vi "TDK 正向工况电流.vi"() -> ()   [LabVIEW 2021]
uses:
  <vilib>/Utility/file.llb/Read Delimited Spreadsheet (DBL).vi
  <instrlib>/TDK-Lambda G Series/TDK-Lambda G Series.lvlib
panel:
  in  "?":enum16{"手动输入", "工况输入"}(ring)
  out "?":bool
  in  "延迟时间":dbl=1.0 caption="延迟时间(s)"
  in  "电流(A)":dbl
  in  "电流方向控制":cluster{"正向":bool, "反向":bool}
  out "工况电流":string[][](table)
  in  "TDK地址":refnum<visa-resource-name>="COM15"
  in  "file path (dialog if empty)":path caption="电流加载"
  in  "电源台数":dbl=3.0
  in  "循环次数":i32
  in  "?":bool
  out "已完成循环次数":i32
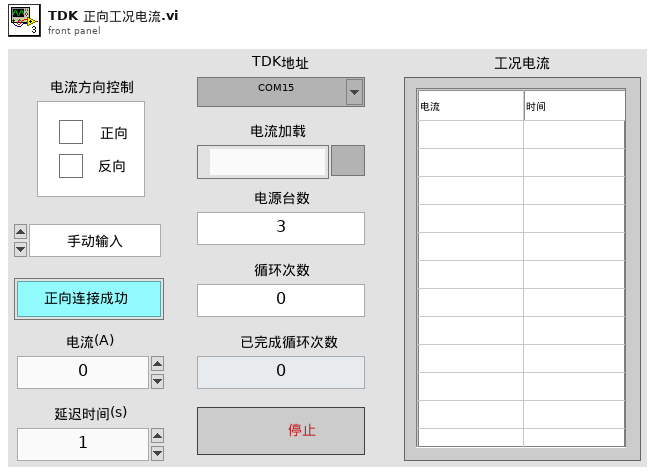
[diagram p1: front panel]
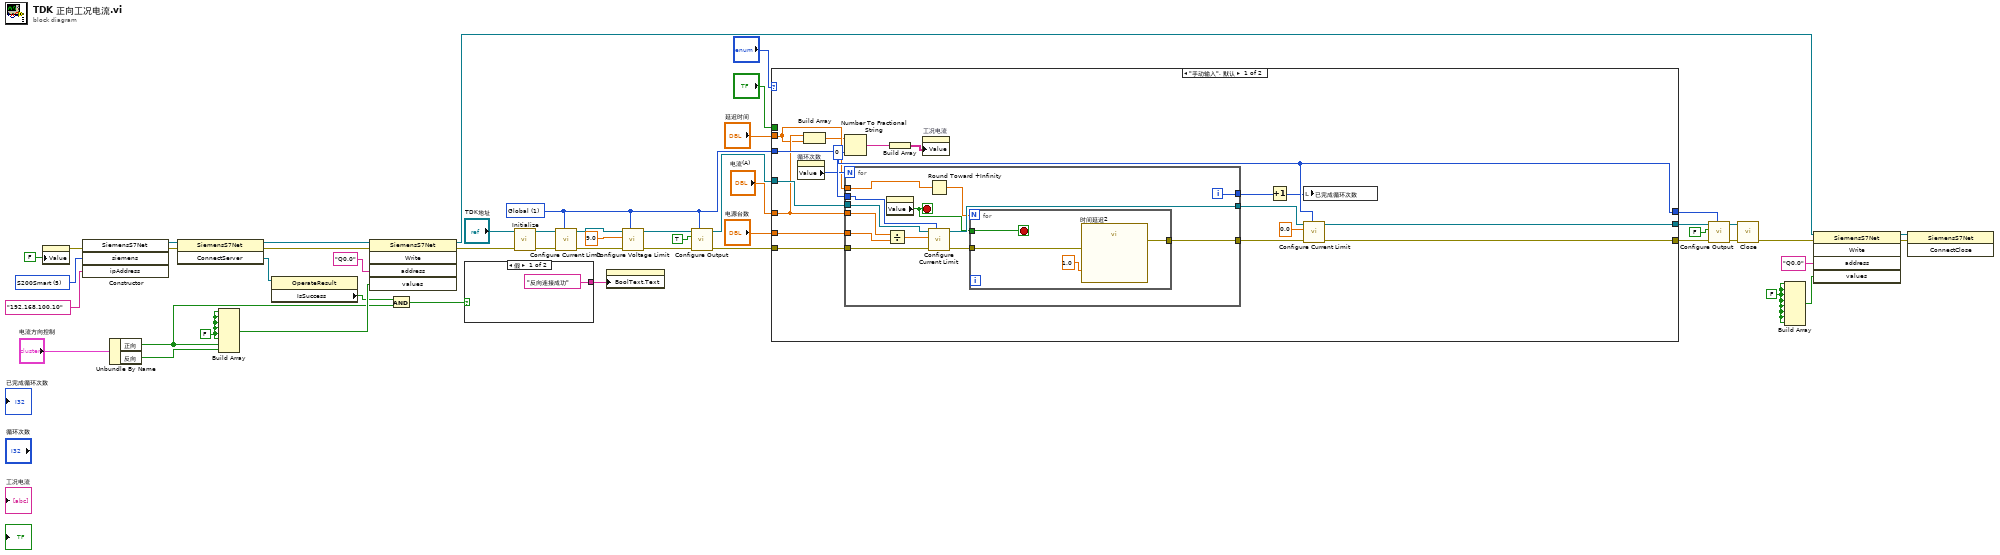
[diagram p0: block diagram]
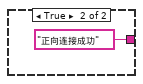
[diagram p2: hidden frame]
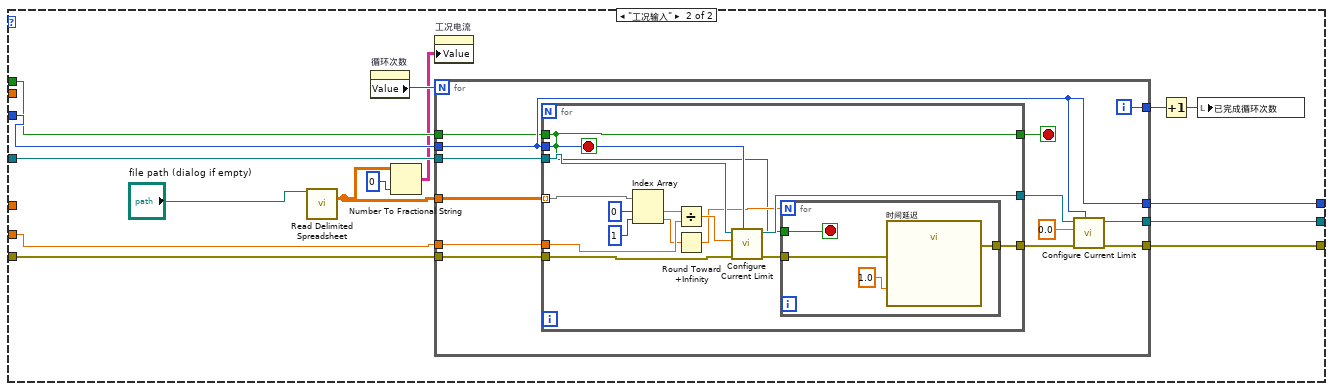
[diagram p3: hidden frame]
diagram:
  w12 = FALSE ("停止")
  w11 = FALSE ("停止")
  w22 = 5 items=["S1200"=1, "S300"=2, "S400"=3, "S1500"=4, "S200Smart"=5, "S200"=6] ("siemens")
  w33 = u16 1 items=["Single", "Global"] ("Globalize (0: Single)")
  n1 = property class="Bool (严格)"("Value"=FALSE ("停止")) -> (error out=w20:errorcluster)  [unwired: 2 in, 1 out]
  n2 = constructor class="SiemensS7Net"(error in=w20, "siemens"=w22, "ipAddress"="192.168.100.10") -> (reference out=w28:refnum<k24>, error out=w29:errorcluster)  [unwired: 2 in, 3 out]
  n3 = Unbundle By Name("电流方向控制") -> ("正向"=w4:bool, "反向"=w2:bool)
  n4 = invoke class="SiemensS7Net" method="ConnectServer"(reference=w28, error in=w29) -> (reference out=w25:refnum<k24>, error out=w24:errorcluster, "ConnectServer"=w27:refnum<k24>)  [unwired: 1 in]
  n5 = Build Array(w11, w11, w11, w11, w11, w11, w4, w2) -> (w23:bool[])
  n6 = property class="OperateResult"(reference=w27) -> ("IsSuccess"=w3:bool)  [unwired: 1 in, 2 out]
  n7 = invoke class="SiemensS7Net" method="Write"(reference=w25, error in=w24, "address"="Q0.0", "values"=w23) -> (reference out=w16:refnum<k24>, error out=w19:errorcluster)  [unwired: 1 in, 3 out]
  n8 = And(x=w3, y=w4) -> (x .and. y?=w1:bool)
  n9 = case shown="假" w1 {
    tunnel: ["反向连接成功" "正向连接成功"] -> w5
    frame False {
    }
    frame True {
    }
  }
  n10 = call <instrlib>:"Initialize.vi"("error in (no error)"=w19, "VISA resource name"="TDK地址") -> ("error out"=w46:errorcluster, "VISA resource name out"=w47:refnum<visa-resource-name>)  [unwired: 8 in]
  n11 = call <instrlib>:"Configure Current Limit.vi"("Globalize (0: Single)"=w33, "error in (no error)"=w46, "VISA resource name"=w47) -> ("error out"=w45:errorcluster, "VISA resource name out"=w44:refnum<visa-resource-name>)  [unwired: 7 in]
  n12 = property class="Bool (严格)"("BoolText.Text"=w5) -> ()  [unwired: 2 in, 2 out]
  n13 = call <instrlib>:"Configure Voltage Limit.vi"("Globalize (0: Single)"=w33, "error in (no error)"=w45, "Voltage Limit (0V)"=9.0 ("Voltage Level (0.0 V)"), "VISA resource name"=w44) -> ("error out"=w39:errorcluster, "VISA resource name out"=w40:refnum<visa-resource-name>)  [unwired: 6 in]
  n14 = call <instrlib>:"Configure Output.vi"("Globalize (0: Single)"=w33, "error in (no error)"=w39, "Enable Output (False)"=TRUE, "VISA resource name"=w40) -> ("error out"=w36:errorcluster, "VISA resource name out"=w37:refnum<visa-resource-name>)  [unwired: 6 in]
  n15 = case shown="\"手动输入\", 默认" "?" {
    tunnel: w37 -> [w69 w101]
    tunnel: w36 -> [w68 w100]
    tunnel: [w64 w99] -> w35
    tunnel: [w63 w98] -> w34
    tunnel: w33 -> [w62 w97]
    tunnel: [w62 w96] -> w32
    tunnel: "电源台数" -> [w59 w93]
    tunnel: "电流(A)" -> [w57 _]
    tunnel: "延迟时间" -> [w56 _]
    tunnel: "?" -> [_ w89]
    frame "手动输入", Default {
      n16 = property on="循环次数" class="DigNum (严格)"() -> ("Value"=w58:i32)  [unwired: 2 in, 2 out]
      n17 = Build Array(w57, w56) -> (w55:dbl[])
      n18 = Number To Fractional String(number=w55, precision (6)=i16 0 ("精度(6)")) -> (F-format string=w54:string[])  [unwired: 2 in]
      n19 = for {
        N: w58 -> [_]
        tunnel: w69 -> [w82]
        tunnel: w68 -> [w81]
        tunnel: [w79] -> w67
        tunnel: [w78] -> w66
        tunnel: w62 -> [w77]
        tunnel: [w75] -> w61
        tunnel: w59 -> [w74]
        tunnel: w57 -> [w73]
        tunnel: w56 -> [w72]
        i -> [w75]
        stop <- w70 stop-if-true
        n20 = property class="Bool (严格)"() -> ("Value"=w70:bool)  [unwired: 2 in, 2 out]
        n21 = Divide(x=w73, y=w74) -> (x/y=w76:dbl)
        n22 = call <instrlib>:"Configure Current Limit.vi"("Globalize (0: Single)"=w77, "error in (no error)"=w81, "Current Limit (0A)"=w76, "VISA resource name"=w82) -> ("error out"=w80:errorcluster, "VISA resource name out"=w78:refnum<visa-resource-name>)  [unwired: 6 in]
        n23 = Round Toward +Infinity(x=w72) -> (ceil(x): smallest int >= x=w71:dbl)
        n24 = for {
          N: w71 -> [_]
          tunnel: w80 -> [w86]
          tunnel: [w85] -> w79
          tunnel: w70 -> [w83]
          stop <- w83 stop-if-true
          n25 = call "时间延迟2"("error in (no error)"=w86, "Delay Time (s)"=1.0) -> ("error out"=w85:errorcluster)  [unwired: 9 in]
        }
      }
      n26 = Build Array(w54) -> (w53:string[][])
      n27 = property on="工况电流" class="Tbl (严格)"("Value"=w53) -> ()  [unwired: 2 in, 2 out]
      n28 = Increment(x=w61) -> (x+1=w60:i32)
      n29 = local write "已完成循环次数"(w60) -> ()
      n30 = call <instrlib>:"Configure Current Limit.vi"("Globalize (0: Single)"=w62, "error in (no error)"=w67, "Current Limit (0A)"=0.0, "VISA resource name"=w66) -> ("error out"=w63:errorcluster, "VISA resource name out"=w64:refnum<visa-resource-name>)  [unwired: 6 in]
    }
    frame "工况输入" {
      n31 = call-poly <vilib>:"Read Delimited Spreadsheet.vi"("file path (dialog if empty)"="file path (dialog if empty)") -> ("all rows"=w91:dbl[][])  [unwired: 9 in, 5 out]
      n32 = property on="循环次数" class="DigNum (严格)"() -> ("Value"=w88:i32)  [unwired: 2 in, 2 out]
      n33 = Number To Fractional String(number=w91, precision (6)=i16 0 ("精度(6)")) -> (F-format string=w87:string[][])  [unwired: 2 in]
      n34 = property on="工况电流" class="Tbl (严格)"("Value"=w87) -> ()  [unwired: 2 in, 2 out]
      n35 = for {
        N: w88 -> [_]
        tunnel: w91 -> [w107]
        tunnel: w97 -> [w106]
        tunnel: [w106] -> w96
        tunnel: [w105] -> w95
        tunnel: w93 -> [w104]
        tunnel: w100 -> [w110]
        tunnel: [w109] -> w98
        tunnel: w101 -> [w112]
        tunnel: [w108] -> w99
        tunnel: w89 -> [w102]
        i -> [w105]
        stop <- w103 stop-if-true
        n36 = for {
          tunnel: w107 -> [w129] mode=indexing
          tunnel: w112 -> [w126]
          tunnel: w110 -> [w125]
          tunnel: [w123] -> w114
          tunnel: [w122] -> w113
          tunnel: w106 -> [w121]
          tunnel: w104 -> [w118]
          tunnel: [w115] -> w103
          tunnel: w102 -> [w115]
          stop <- w115 stop-if-true
          n37 = Index Array(array=w129, index #1=0 ("索引"), index #2=1 ("索引")) -> (element #1=w120:dbl, element #2=w117:dbl)
          n38 = Divide(x=w120, y=w118) -> (x/y=w119:dbl)
          n39 = Round Toward +Infinity(x=w117) -> (ceil(x): smallest int >= x=w116:dbl)
          n40 = call <instrlib>:"Configure Current Limit.vi"("Globalize (0: Single)"=w121, "error in (no error)"=w125, "Current Limit (0A)"=w119, "VISA resource name"=w126) -> ("error out"=w124:errorcluster, "VISA resource name out"=w122:refnum<visa-resource-name>)  [unwired: 6 in]
          n41 = for {
            N: w116 -> [_]
            tunnel: w124 -> [w133]
            tunnel: [w132] -> w123
            tunnel: w115 -> [w130]
            stop <- w130 stop-if-true
            n42 = call "时间延迟"("error in (no error)"=w133, "Delay Time (s)"=1.0) -> ("error out"=w132:errorcluster)  [unwired: 9 in]
          }
        }
        n43 = call <instrlib>:"Configure Current Limit.vi"("Globalize (0: Single)"=w106, "error in (no error)"=w114, "Current Limit (0A)"=0.0, "VISA resource name"=w113) -> ("error out"=w109:errorcluster, "VISA resource name out"=w108:refnum<visa-resource-name>)  [unwired: 6 in]
      }
      n44 = Increment(x=w95) -> (x+1=w94:i32)
      n45 = local write "已完成循环次数"(w94) -> ()
    }
  }
  n46 = call <instrlib>:"Configure Output.vi"("Globalize (0: Single)"=w32, "error in (no error)"=w34, "Enable Output (False)"=FALSE ("Enable Output (True)"), "VISA resource name"=w35) -> ("error out"=w41:errorcluster, "VISA resource name out"=w42:refnum<visa-resource-name>)  [unwired: 6 in]
  n47 = call <instrlib>:"Close.vi"("error in (no error)"=w41, "VISA resource name"=w42) -> ("error out"=w14:errorcluster)  [unwired: 9 in]
  n48 = Build Array(w12, w12, w12, w12, w12, w12, w12, w12) -> (w17:bool[])
  n49 = invoke class="SiemensS7Net" method="Write"(reference=w16, error in=w14, "address"="Q0.0", "values"=w17) -> (reference out=w15:refnum<k24>, error out=w13:errorcluster)  [unwired: 1 in, 3 out]
  n50 = invoke class="SiemensS7Net" method="ConnectClose"(reference=w15, error in=w13) -> ()  [unwired: 1 in, 3 out]
